vi "Take Step.vi"(8 "error in (no error)":errorcluster, 10 "Maze In":refnum<class "Maze.lvclass">, 11 "Mouse in":refnum<class "Mouse.lvclass">) -> (0 "error out":errorcluster, 2 "Maze":refnum<class "Maze.lvclass">, 3 "Mouse out":refnum<class "Mouse.lvclass">, 5 "Move?":bool, 7 "Crash?":bool)   [LabVIEW 2020, in "Maze.lvlib" / "Mouse.lvclass"]
doc: "Takes a step for the mouse instance. Calls the child implementation's Decide Action and then updates the state to reflect that choice. Checks for wall crashes to ensure implementations are monitoring distances properly."
uses:
  Mouse.lvclass
  Maze/Maze.lvclass
  Mouse.lvclass/Mouse.ctl
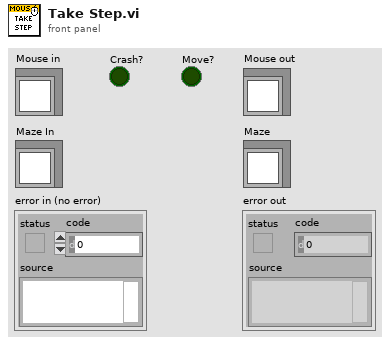
[diagram p1: front panel]
types:
  T1 = typedef "Maze.lvlib/Action.ctl" = enum16{"Turn Left", "Turn Right", "Forward"}
  T2 = typedef "Maze.lvlib/Direction.ctl" = enum8{"East", "North", "West", "South"}
  T3 = typedef "Maze.lvlib/Position.ctl" = cluster{"S":i32, "E":i32}
  T4 = typedef "Maze.lvlib/Adjacency.ctl" = cluster{"E":bool, "N":bool, "W":bool, "S":bool, "Goal":bool, "Start":bool}
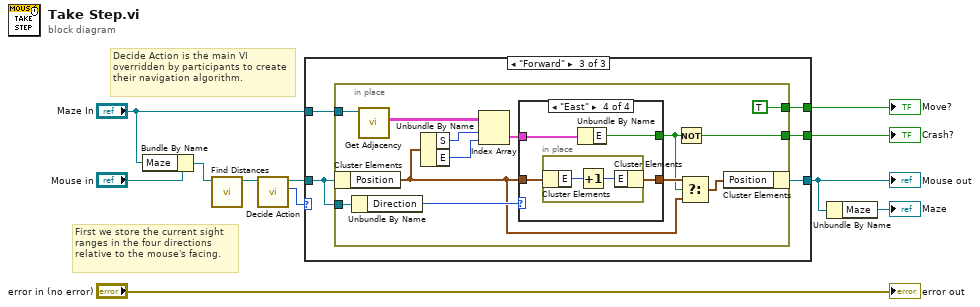
[diagram p0: block diagram]
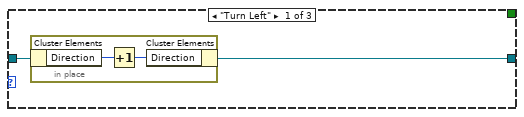
[diagram p2: hidden frame]
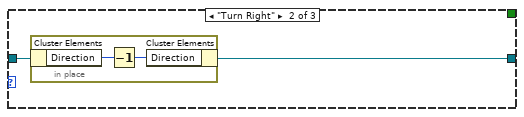
[diagram p3: hidden frame]
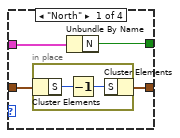
[diagram p4: hidden frame]
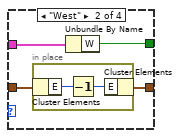
[diagram p5: hidden frame]
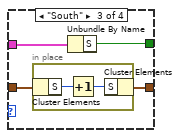
[diagram p6: hidden frame]
diagram:
  # "Decide Action is the main VI overridden by participants to create their navigation algorithm."
  # "First we store the current sight ranges in the four directions relative to the mouse's facing."
  n1 = Bundle By Name(cluster="Mouse in", "Maze"="Maze In") -> (w4:refnum<class "Mouse.lvclass">)
  n2 = call "Find Distances.vi"("Mouse in"=w4) -> ("Mouse out"=w10:refnum<class "Mouse.lvclass">)  [unwired: 10 in]
  n3 = call-dynamic "Decide Action.vi"("Mouse in"=w10) -> ("Action"=w9:T1, "Mouse out"=w8:refnum<class "Mouse.lvclass">)  [unwired: 8 in, 1 out]
  n4 = case shown="\"Forward\"" w9 {
    tunnel: w8 -> [w13 w17 w24]
    tunnel: [w12 w16 w21] -> w2
    tunnel: "Maze In" -> [_ _ w23]
    tunnel: [_ _ w22] -> w7
    tunnel: [_ _ w20] -> w6
    frame "Turn Left" {
      n5 = in-place {
        n6 = in-place-cluster #1(w13) -> ("Direction"=w15:T2)
        n7 = Increment(x=w15) -> (x+1=w14:T2)
        n8 = in-place-cluster #1("Direction"=w14) -> (w12:refnum<class "Mouse.lvclass">)
      }
    }
    frame "Turn Right" {
      n9 = in-place {
        n10 = in-place-cluster #2(w17) -> ("Direction"=w19:T2)
        n11 = Decrement(x=w19) -> (x-1=w18:T2)
        n12 = in-place-cluster #2("Direction"=w18) -> (w16:refnum<class "Mouse.lvclass">)
      }
    }
    frame "Forward" {
      n13 = in-place {
        in-place-border: w24 -> [w37]
        in-place-border: w23 -> [w36]
        in-place-border: [w26] -> w22
        in-place-border: [TRUE] -> w20
        n14 = in-place-cluster #3(w24) -> ("Position"=w29:T3)
        n15 = Unbundle By Name(w37) -> ("Direction"=w31:T2)
        n16 = call "Get Adjacency.vi"("Maze in"=w36) -> ("Adjacency"=w35:T4[][])  [unwired: 8 in, 2 out]
        n17 = Unbundle By Name(w29) -> ("S"=w33:i32, "E"=w34:i32)
        n18 = Index Array(array=w35, index (row)=w33, index (col)=w34) -> (element=w32:T4)
        n19 = case shown="\"East\"" w31 {
          tunnel: w32 -> [w39 w45 w51 w57]
          tunnel: w29 -> [w41 w47 w53 w59]
          tunnel: [w40 w46 w52 w58] -> w30
          tunnel: [w38 w44 w50 w56] -> w27
          frame "North" {
            n20 = in-place {
              n21 = in-place-cluster #4(w41) -> ("S"=w43:i32)
              n22 = Decrement(x=w43) -> (x-1=w42:i32)
              n23 = in-place-cluster #4("S"=w42) -> (w40:T3)
            }
            n24 = Unbundle By Name(w39) -> ("N"=w38:bool)
          }
          frame "West" {
            n25 = in-place {
              n26 = in-place-cluster #5(w47) -> ("E"=w49:i32)
              n27 = Decrement(x=w49) -> (x-1=w48:i32)
              n28 = in-place-cluster #5("E"=w48) -> (w46:T3)
            }
            n29 = Unbundle By Name(w45) -> ("W"=w44:bool)
          }
          frame "South" {
            n30 = in-place {
              n31 = in-place-cluster #6(w53) -> ("S"=w55:i32)
              n32 = Increment(x=w55) -> (x+1=w54:i32)
              n33 = in-place-cluster #6("S"=w54) -> (w52:T3)
            }
            n34 = Unbundle By Name(w51) -> ("S"=w50:bool)
          }
          frame "East" {
            n35 = in-place {
              n36 = in-place-cluster #7(w59) -> ("E"=w61:i32)
              n37 = Increment(x=w61) -> (x+1=w60:i32)
              n38 = in-place-cluster #7("E"=w60) -> (w58:T3)
            }
            n39 = Unbundle By Name(w57) -> ("E"=w56:bool)
          }
        }
        n40 = Not(x=w27) -> (.not. x?=w26:bool)
        n41 = Select(t=w30, s=w27, f=w29) -> (s? t:f=w28:T3)
        n42 = in-place-cluster #3("Position"=w28) -> (w21:refnum<class "Mouse.lvclass">)
      }
    }
  }
  "Mouse out" <- w2
  "Crash?" <- w7
  "Move?" <- w6
  n43 = Unbundle By Name(w2) -> ("Maze"=→"Maze":refnum<class "Maze.lvclass">)
  "error out" <- "error in (no error)"
